vi "LIA Power Spectrum.vi"(10 "waveform":waveform(cdb), 11 "window":T1 items=["Rectangle"=0, "Hanning"=1, "Hamming"=2, "Blackman-Harris"=3, "Exact Blackman"=4, "Blackman"=5, "Flat Top"=6, "4 Term B-Harris "=7, "7 Term B-Harris"=8, "Low Sidelobe"=9, "Blackman Nuttall"=11, "Triangle"=30, "Bartlett-Hanning"=31, "Bohman"=32, "Parzen"=33, "Welch"=34, "Kaiser"=60, "Dolph-Chebyshev"=61, "Gaussian"=62]) -> (3 "Waveform Graph 5":cluster{"x0":dbl, "dx":dbl, "Y":dbl[]})   [LabVIEW 2017]
uses:
  <vilib>/Analysis/4window.llb/windowTd.ctl
  <vilib>/Analysis/2dsp.llb/Complex FFT.vi
  <vilib>/Analysis/0measdsp.llb/Scaled Time Domain Window (CDB).vi
  <vilib>/measure/NI_MAPro.lvlib
  <vilib>/Analysis/NI_AALPro.lvlib
  <vilib>/measure/maspectr.llb/FFT Power Spectrum and PSD for 1 Chan (CDB).vi
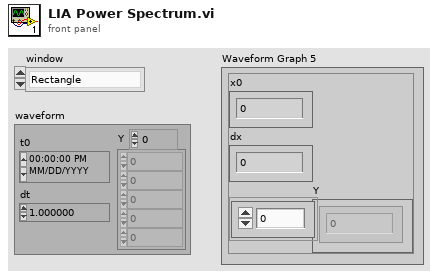
[diagram p1: front panel]
types:
  T1 = typedef "NI_AALPro.lvlib/windowTd.ctl" = u32
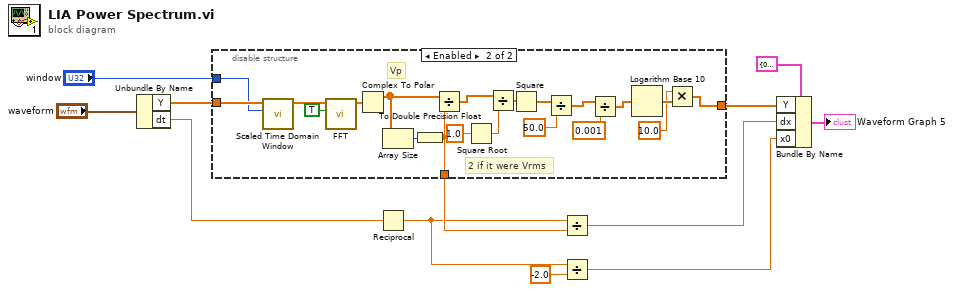
[diagram p0: block diagram]
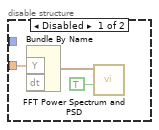
[diagram p2: hidden frame]
diagram:
  n1 = Unbundle By Name("waveform") -> ("Y"=w5:cdb[], "dt"=w8:dbl)
  n2 = disable-structure shown="Enabled" {
    disable-tunnel: w5 -> [w15 w21]
    disable-tunnel: [_ w16] -> w7
    disable-tunnel: [_ w19] -> w10
    disable-tunnel: "window" -> [_ w18]
    frame Disabled {
      n3 = Bundle By Name("Y"=w15) -> (w14:waveform(cdb))  [unwired: 2 in]
      n4 = call-poly <vilib>:"FFT Power Spectrum and PSD.vi"("dB On (F)"=TRUE, "time signal"=w14) -> ()  [unwired: 6 in, 4 out]
    }
    frame Enabled {
      # "2 if it were Vrms"
      # "Vp"
      n5 = call-poly <vilib>:"Scaled Time Domain Window.vi"("window"=w18, "X"=w21) -> ("Windowed X"=w20:cdb[])  [unwired: 7 in, 2 out]
      n6 = call-poly <vilib>:"FFT.vi"("shift?"=TRUE, "X"=w20) -> ("FFT {X}"=w35:cdb[])  [unwired: 8 in, 1 out]
      n7 = Complex To Polar(r * e^(i*theta)=w35) -> (r=w34:dbl[])  [unwired: 1 out]
      n8 = Array Size(array=w34) -> (size(s)=w33:i32)
      n9 = To Double Precision Float(number=w33) -> (double precision float=w19:dbl)
      n10 = Divide(x=w34, y=w19) -> (x/y=w17:dbl[])
      n11 = Square Root(x=1.0) -> (sqrt(x)=w24:dbl)
      n12 = Divide(x=w17, y=w24) -> (x/y=w22:dbl[])
      n13 = Square(x=w22) -> (x^2=w32:dbl[])
      n14 = Divide(x=w32, y=50.0) -> (x/y=w28:dbl[])
      n15 = Divide(x=w28, y=0.001) -> (x/y=w23:dbl[])
      n16 = Logarithm Base 10(1:w23) -> (0:w30:dbl[])
      n17 = Multiply(x=10.0, y=w30) -> (x*y=w16:dbl[])
    }
  }
  n18 = Reciprocal(x=w8) -> (1/x=w3:dbl)
  n19 = Divide(x=w3, y=w10) -> (x/y=w9:dbl)
  n20 = Divide(x=w3, y=-2.0) -> (x/y=w1:dbl)
  n21 = Bundle By Name(cluster=cluster{"x0":dbl, "dx":dbl, "Y":dbl[]} {"x0"=0.0, "dx"=1.0, "Y"=[]} ("Waveform Graph 5"), "Y"=w7, "dx"=w9, "x0"=w1) -> (→"Waveform Graph 5":cluster{"x0":dbl, "dx":dbl, "Y":dbl[]})
